vi "DDAQ-Get.vi"(8 "error in (no error)":errorcluster, 9 "max bytes to read (10000)":i32=10000, 10 "SCPI-like Keyword (leave off question mark)":string, 11 "connection ID":refnum<k5>) -> (0 "error out":errorcluster, 1 "Query":string, 2 "Response":string, 3 "connection ID out":refnum<k5>)   [LabVIEW 2020]
panel:
  out "Response (as number)":dbl
  out "bytes written":i32
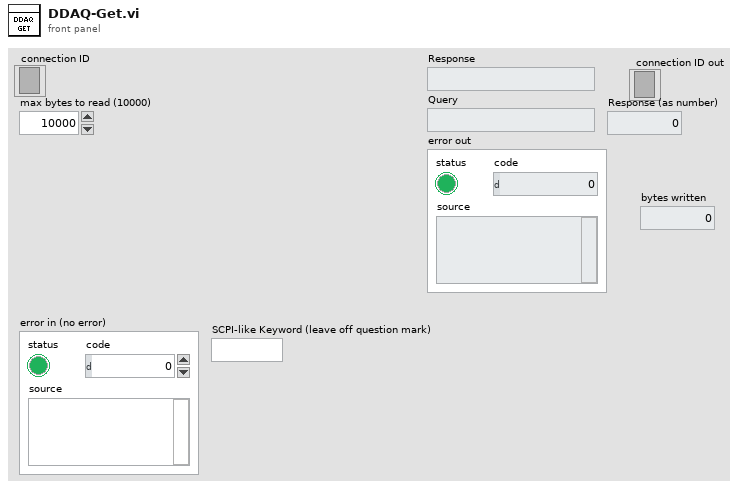
[diagram p1: front panel]
types:
  T1 = enum16{"Standard", "Buffered", "CRLF", "Immediate"}
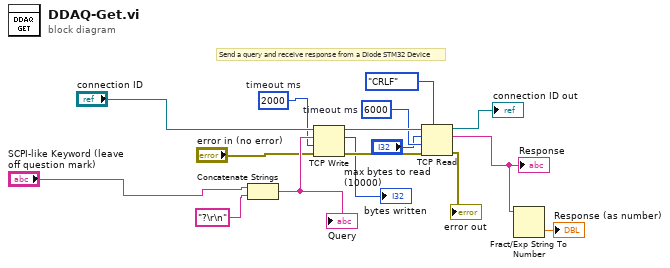
[diagram p0: block diagram]
diagram:
  w3 = 6000  # timeout ms
  w4 = 2000  # timeout ms
  # "Send a query and receive response from a Diode STM32 Device"
  n1 = Concatenate Strings("SCPI-like Keyword (leave off question mark)", "?\r\n") -> (w14:string)
  "Query" <- w14
  n2 = TCP Write(connection ID="connection ID", data in=w14, error in (no error)="error in (no error)", 9:w4) -> (connection ID out=w12:refnum<k5>, bytes written=→"bytes written":i32, error out=w11:errorcluster)
  n3 = TCP Read(connection ID=w12, bytes to read="max bytes to read (10000)", error in (no error)=w11, 7:T1."CRLF" ("mode (standard)"), 9:w3) -> (connection ID out=→"connection ID out":refnum<k5>, data out=w6:string, error out=→"error out":errorcluster)
  "Response" <- w6
  n4 = Fract/Exp String To Number(string=w6) -> (number=→"Response (as number)":dbl)  [unwired: 3 in, 1 out]
